vi "GroundPassWrapper.vi"(7 "State":T1, 8 "error in":errorcluster) -> (0 "error out":errorcluster)   [LabVIEW 2013]
uses:
  PassState.ctl
  DoubleSolenoidAction.ctl
  RollerAction.ctl
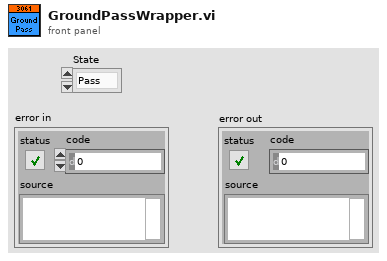
[diagram p1: front panel]
types:
  T1 = typedef "PassState.ctl" = enum16{"Pass", "Stop"}
  T2 = typedef "DoubleSolenoidAction.ctl" = enum16{"Init", "Middle", "In", "Out"}
  T3 = typedef "RollerAction.ctl" = enum16{"Init", "Off", "Forward", "Reverse"}
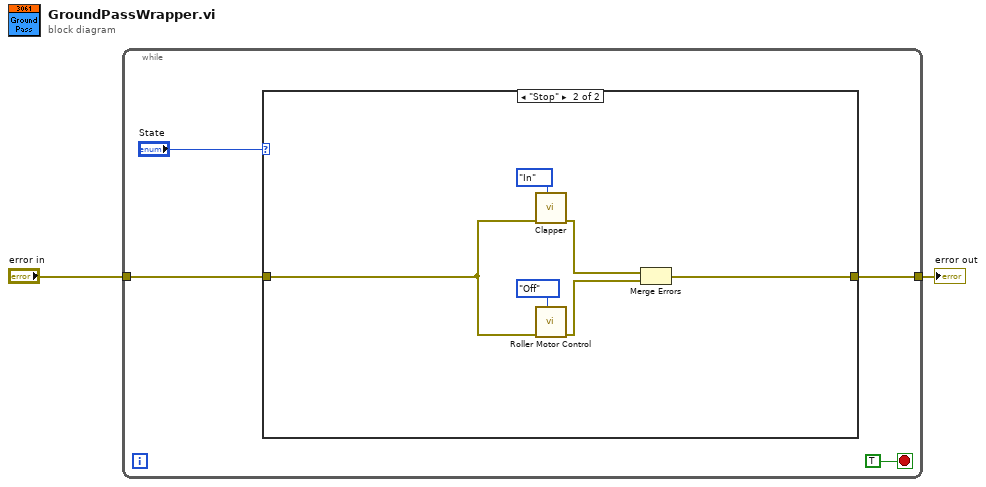
[diagram p0: block diagram]
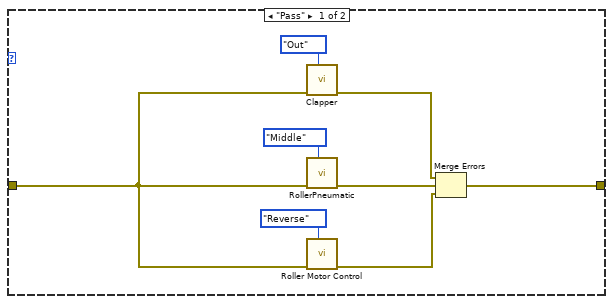
[diagram p2: hidden frame]
diagram:
  n1 = while {
    tunnel: "error in" -> [w5]
    tunnel: [w4] -> w1
    stop <- TRUE stop-if-true
    n2 = case shown="\"Stop\"" "State" {
      tunnel: w5 -> [w11 w18]
      tunnel: [w7 w15] -> w4
      frame "Pass" {
        n3 = call "Clapper.vi"("State"=DoubleSolenoidAction."Out", "Error in"=w11) -> ("Error out"=w10:errorcluster)  [unwired: 9 in]
        n4 = call "RollerPneumatic.vi"("State"=DoubleSolenoidAction."Middle", "Error in"=w11) -> ("Error out"=w9:errorcluster)  [unwired: 9 in]
        n5 = call "Roller Motor Control.vi"("Action"=RollerAction."Reverse", "Error in"=w11) -> ("Error out"=w8:errorcluster)  [unwired: 9 in]
        n6 = Merge Errors(w10, w9, w8) -> (w7:errorcluster)
      }
      frame "Stop" {
        n7 = call "Clapper.vi"("State"=DoubleSolenoidAction."In", "Error in"=w18) -> ("Error out"=w17:errorcluster)  [unwired: 9 in]
        n8 = call "Roller Motor Control.vi"("Action"=RollerAction."Off", "Error in"=w18) -> ("Error out"=w16:errorcluster)  [unwired: 9 in]
        n9 = Merge Errors(w17, w16) -> (w15:errorcluster)
      }
    }
  }
  "error out" <- w1
